vi "Read left SR.vi"(9 "ShiftRegister in":refnum<class "ShiftRegister.lvclass">) -> (3 "ShiftRegister out":refnum<class "ShiftRegister.lvclass">, 4 "left SR":refnum<class "LeftShiftRegister.lvclass">[](array[class]))   [LabVIEW 2014, in "ShiftRegister.lvclass"]
uses:
  ShiftRegister.lvclass
  LeftShiftRegister/LeftShiftRegister.lvclass
  ShiftRegister.lvclass/ShiftRegister.ctl
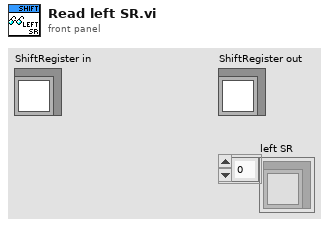
[diagram p1: front panel]
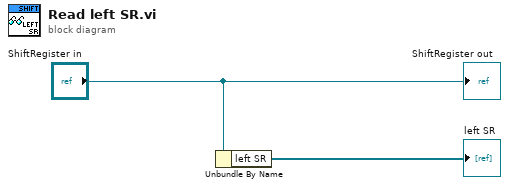
[diagram p0: block diagram]
diagram:
  n1 = Unbundle By Name("ShiftRegister in") -> ("left SR"=→"left SR":refnum<class "LeftShiftRegister.lvclass">[])
  "ShiftRegister out" <- "ShiftRegister in"
